vi "niRFUtil FTW FFT.vi"   [LabVIEW 2015, in "niRFUtil.lvlib"]
doc: "(c) Copyright 2006, National Instruments, Inc. This VI may not be duplicated, sold, or distributed without written consent from National Instruments."
uses:
  niRFUtil.lvlib
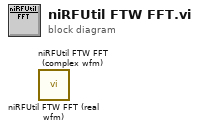
[diagram p0: block diagram]
diagram:
  n1 = call "niRFUtil FTW FFT (real wfm).vi"() -> ()  [unwired: 3 in, 3 out]
  n2 = call "niRFUtil FTW FFT (complex wfm).vi"() -> ()  [unwired: 3 in, 3 out]
